vi "TAI_Motor.vi"(3 "Normal Output":dbl, 4 "Aux Trigger":bool, 5 "Override Actuator Bypass":bool, 6 "Actuator Name":string) -> (0 "Interlocked Output":dbl, 2 "Output Mode":T1(ring))   [LabVIEW 2020]
doc: "This VI is configured for polymorphic use and functions as an interlock, allowing the selected motor to be tested manually via the FRC 4265 Dashboard. During testing, all interlocked actuators which are not selected for testing are disabled."
uses:
  b41506b6-27dc-4ca7-820b-83b05fbff20d.vi
  ce8c15ce-250d-419c-a833-6f2ecce11d20.vi
  GlobalDriverStationData.vi
  Timer.vi
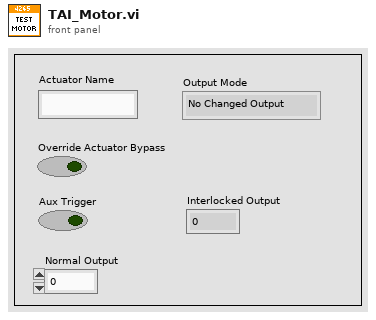
[diagram p1: front panel]
types:
  T1 = enum16{"No Changed Output", "New Normal Output", "New Testing Output"}
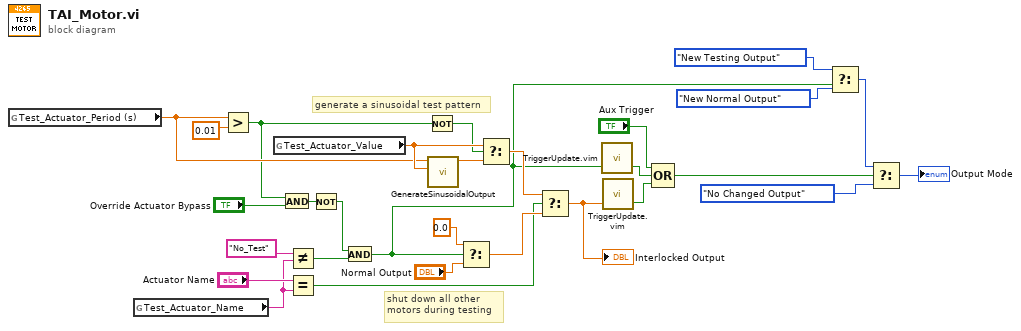
[diagram p0: block diagram]
diagram:
  # "generate a sinusoidal test pattern"
  # "shut down all other\nmotors during testing"
  n1 = global read "GlobalDriverStationData.vi" "Test_Actuator_Period (s)"() -> (w20:dbl)
  n2 = global read "GlobalDriverStationData.vi" "Test_Actuator_Name"() -> (w24:string)
  n3 = Greater?(x=w20, y=0.01) -> (0:w16:bool)
  n4 = global read "GlobalDriverStationData.vi" "Test_Actuator_Value"() -> (w21:dbl)
  n5 = And(x=w16, y="Override Actuator Bypass") -> (x .and. y?=w14:bool)
  n6 = Not Equal?(x="No_Test", y=w24) -> (x != y?=w18:bool)
  n7 = Equal?(x="Actuator Name", y=w24) -> (x = y?=w6:bool)
  n8 = Not(x=w14) -> (.not. x?=w17:bool)
  n9 = And(x=w17, y=w18) -> (x .and. y?=w2:bool)
  n10 = Not(x=w16) -> (.not. x?=w13:bool)
  n11 = call "GenerateSinusoidalOutput.vi"("Amplitude"=w21, "Period (s)"=w20) -> ("sin(time)"=w23:dbl)  [unwired: 9 in]
  n12 = Select(t=0.0, s=w2, f="Normal Output") -> (s? t:f=w25:dbl)
  n13 = Select(t=w21, s=w13, f=w23) -> (s? t:f=w22:dbl)
  n14 = Select(t=w22, s=w6, f=w25) -> (s? t:f=w12:dbl)
  "Interlocked Output" <- w12
  n15 = call "TriggerUpdate.vim"("Trigger"=w2) -> ("Update"=w5:bool)  [unwired: 2 in]
  n16 = call "TriggerUpdate.vim"("Trigger"=w12) -> ("Update"=w4:bool)  [unwired: 2 in]
  n17 = Compound Arithmetic op=OR("Aux Trigger", w5, w4) -> (w3:bool)
  n18 = Select(t=T1."New Testing Output", s=w2, f=T1."New Normal Output") -> (s? t:f=w9:T1)
  n19 = Select(t=w9, s=w3, f=T1."No Changed Output") -> (s? t:f=→"Output Mode":T1)
